vi "Read ID.vi"(8 "error in (no error)":errorcluster, 11 "Alicat Data in":refnum<class "Alicat Data.lvclass">) -> (0 "error out":errorcluster, 2 "ID":string, 3 "Alicat Data out":refnum<class "Alicat Data.lvclass">)   [LabVIEW 2015, in "Alicat Lib.lvlib" / "Alicat Data.lvclass"]
uses:
  Alicat Data.lvclass
  Alicat Data.lvclass/Alicat Data.ctl
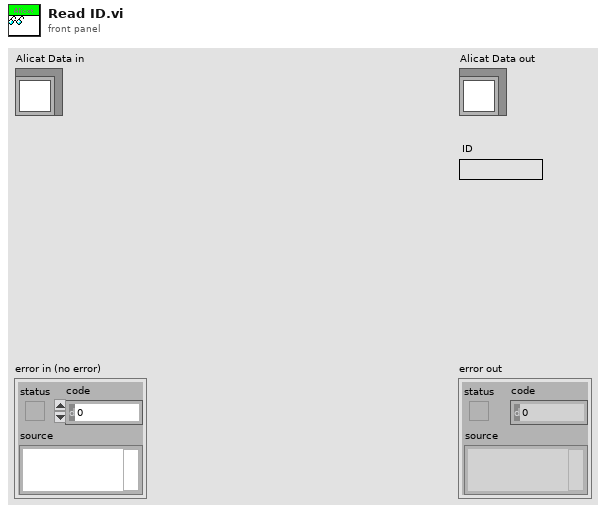
[diagram p1: front panel]
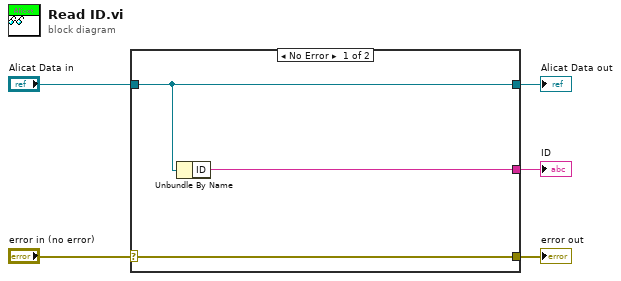
[diagram p0: block diagram]
diagram:
  n1 = case shown="No Error" "error in (no error)" {
    selector: "error in (no error)" -> [w8 w9]
    tunnel: [w8 w9] -> w4
    tunnel: [w7 w10] -> w2
    tunnel: "Alicat Data in" -> [w7 w10]
    tunnel: [w6 _] -> w1
    frame No Error {
      n2 = Unbundle By Name(w7) -> ("ID"=w6:string)
    }
    frame Error {
    }
  }
  "error out" <- w4
  "Alicat Data out" <- w2
  "ID" <- w1
